vi "String to JSON String.vi"(8 "error in (no error)":errorcluster, 11 "String":string) -> (0 "error out":errorcluster, 3 "String for JSON":string)   [LabVIEW 2021, in "DataTypes_CIF_U.lvlib"]
doc: "Embedding a string in JSON requires additional formatting. This will reformat so it can be embedded as part of a JSON message."
uses:
  DataTypes_CIF_U.lvlib
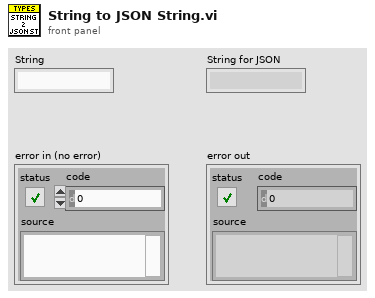
[diagram p1: front panel]
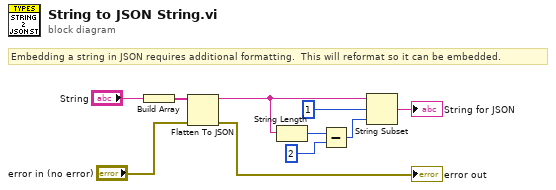
[diagram p0: block diagram]
diagram:
  # "Embedding a string in JSON requires additional formatting.  This will reformat so it can be embedded."
  n1 = Build Array("String") -> (w10:string[])
  n2 = Flatten To JSON(anything=w10, error in (no error)="error in (no error)") -> (JSON string=w7:string, 11:→"error out":errorcluster)  [unwired: 1 in]
  n3 = String Length(string=w7) -> (length=w9:i32)
  n4 = Subtract(x=w9, y=2 ("2")) -> (x-y=w6:i32)
  n5 = String Subset(string=w7, offset (0)=1, length (rest)=w6) -> (substring=→"String for JSON":string)
